vi "emi_Deg to Rad.vi"(7 "Deg":dbl) -> (8 "Rad":dbl)   [LabVIEW 2010]
doc: "Convert a double containgng an angle in degrees, to an angle in radiance."
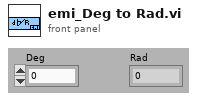
[diagram p1: front panel]
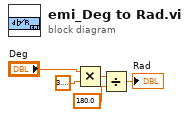
[diagram p0: block diagram]
diagram:
  n1 = Multiply(x="Deg", y=3.141592653589793) -> (x*y=w3:dbl)
  n2 = Divide(x=w3, y=180.0) -> (x/y=→"Rad":dbl)
